vi "determineCommonBaseConfigPath.vi"(8 "error in (no error)":errorcluster, 11 "ConfigurationFileReader in":refnum<class "ConfigurationFileReader.lvclass">) -> (0 "error out":errorcluster, 2 "ConfigurationPath":path, 3 "ConfigurationFileReader out":refnum<class "ConfigurationFileReader.lvclass">)   [LabVIEW 2016, in "Settings.lvlib" / "ConfigurationFileReader.lvclass"]
uses:
  ConfigurationFileReader.lvclass
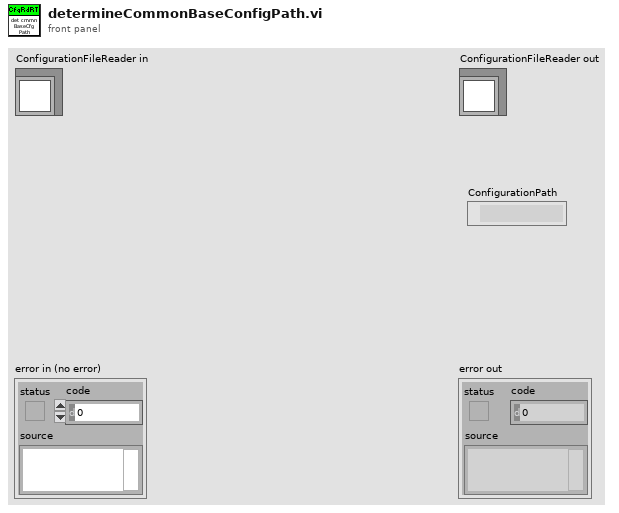
[diagram p1: front panel]
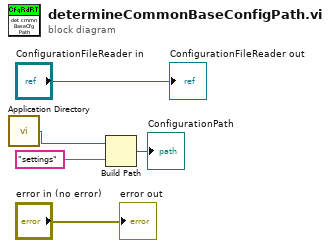
[diagram p0: block diagram]
diagram:
  n1 = call <vilib>:"Application Directory.vi"() -> ("Application Directory"=w1:path)
  n2 = Build Path(base path=w1, name or relative path="settings") -> (appended path=→"ConfigurationPath":path)
  "error out" <- "error in (no error)"
  "ConfigurationFileReader out" <- "ConfigurationFileReader in"
